vi "Configure.vi"(8 "error in (no error)":errorcluster, 9 "Resolution":enum16{"5 1/2 Digits", "6 1/2 Digits"}(ring), 10 "Range":enum16{"1V", "10V", "100V"}(ring), 11 "DMM_Concrete in":refnum<class "DMM_Concrete.lvclass">) -> (0 "error out":errorcluster, 3 "DMM_Concrete out":refnum<class "DMM_Concrete.lvclass">)   [LabVIEW 2024, in "HAL_Example.lvlib" / "DMM_Concrete.lvclass"]
uses:
  DMM/DMM_Concrete.lvclass
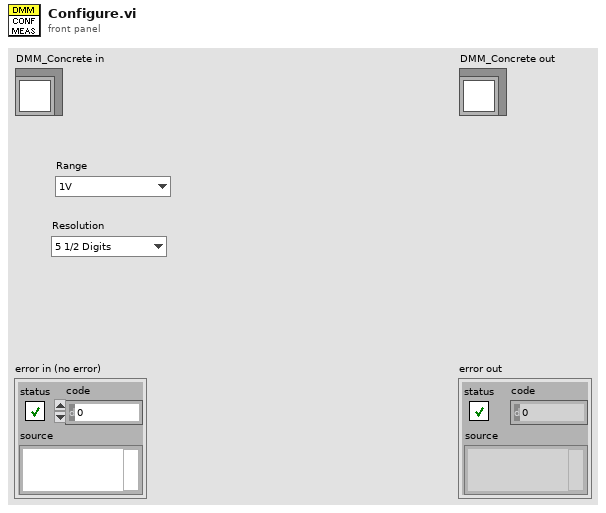
[diagram p1: front panel]
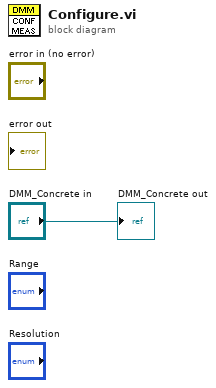
[diagram p0: block diagram]
diagram:
  "DMM_Concrete out" <- "DMM_Concrete in"
